vi "Init Table Data.vi"(8 "error in (no error)":errorcluster, 10 "Item Names":string[][](array[string]), 11 "Table":refnum<vi>) -> (0 "error out":errorcluster)   [LabVIEW 2016, in "System Mapping Tool.lvlib"]
uses:
  System Mapping Tool.lvlib
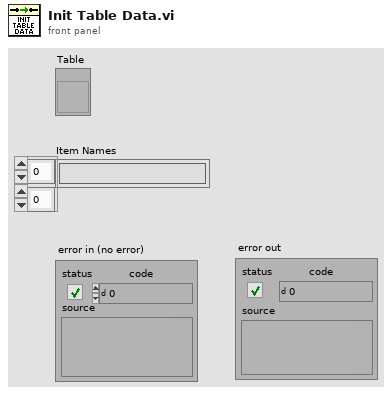
[diagram p1: front panel]
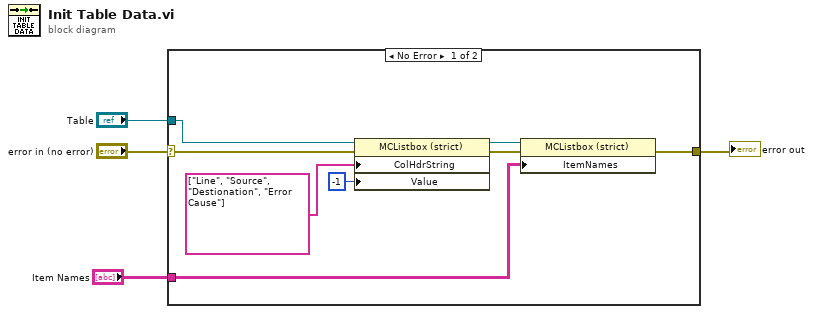
[diagram p0: block diagram]
diagram:
  n1 = case shown="No Error" "error in (no error)" {
    selector: "error in (no error)" -> [w10 w13]
    tunnel: [w9 w13] -> w3
    tunnel: "Item Names" -> [w7 _]
    tunnel: "Table" -> [w6 _]
    frame No Error {
      n2 = property class="MCListbox (strict)"(reference=w6, error in=w10, "ColHdrString"=string[] ["Line", "Source", "Destionation", "Error Cause"] ("Column Header Strings[]"), "Value"=-1) -> (reference out=w11:refnum<vi>, error out=w12:errorcluster)
      n3 = property class="MCListbox (strict)"(reference=w11, error in=w12, "ItemNames"=w7) -> (error out=w9:errorcluster)  [unwired: 1 out]
    }
    frame Error {
    }
  }
  "error out" <- w3
